vi "stopHandler.vi"(9 "stopOperationalMode":bool, 10 "stopVoltageAlert":bool, 11 "stopMain":bool) -> (2 "stop":bool)   [LabVIEW 2014]
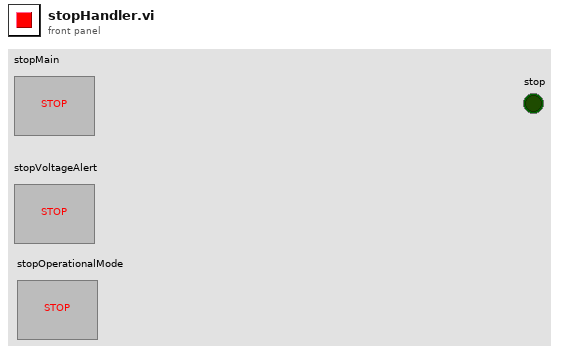
[diagram p1: front panel]
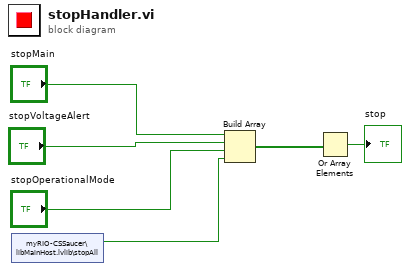
[diagram p0: block diagram]
diagram:
  n1 = shared-variable "myRIO-CSSaucer\\libMainHost.lvlib\\stopAll"() -> (w1:bool)  [unwired: 1 in, 1 out]
  n2 = Build Array("stopMain", "stopVoltageAlert", "stopOperationalMode", w1) -> (w3:bool[])
  n3 = Or Array Elements(Boolean array=w3) -> (logical OR=→"stop":bool)
